vi "Run.vi"(8 "error in (no error)":errorcluster, 11 "TCS in":refnum<class "TCS.lvclass">) -> (0 "error out":errorcluster, 3 "TCS out":refnum<class "TCS.lvclass">)   [LabVIEW 2018, in "TCS.lvclass"]
uses:
  TCS.lvclass
  TCS.lvclass/TCS.ctl
  State Machine/State Machine.lvclass/State Machine.ctl
  State Machine/State Machine.lvclass
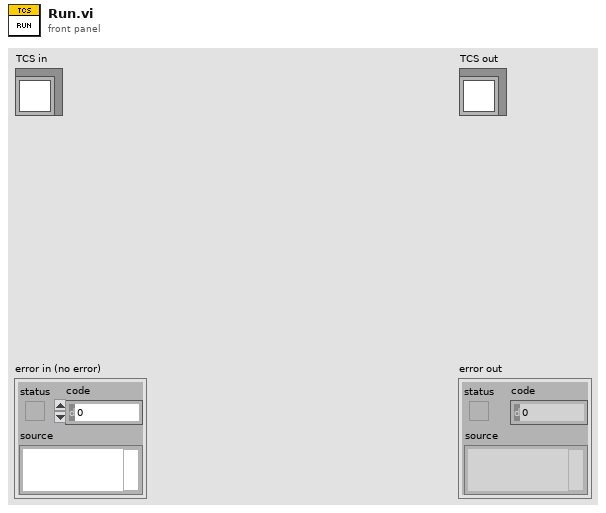
[diagram p1: front panel]
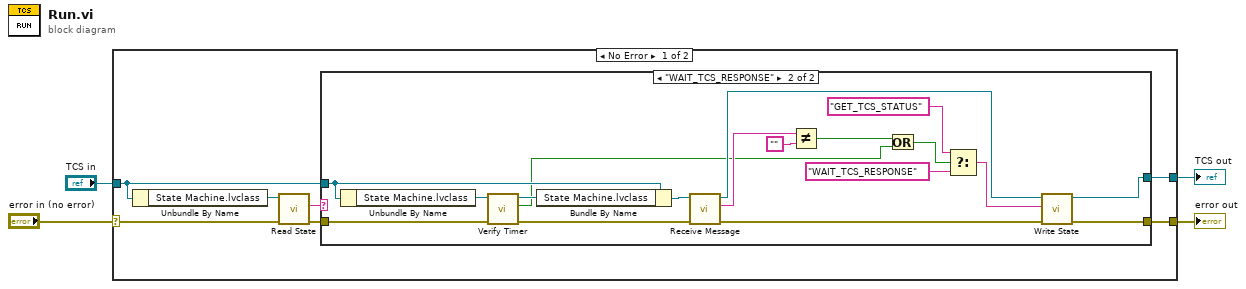
[diagram p0: block diagram]
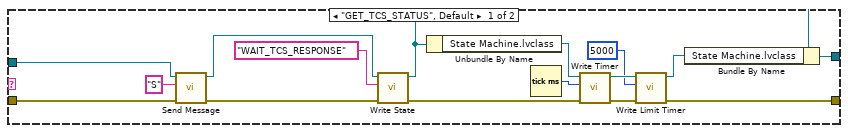
[diagram p2: hidden frame]
diagram:
  n1 = case shown="No Error" "error in (no error)" {
    selector: "error in (no error)" -> [w10 w47]
    tunnel: [w5 w47] -> w3
    tunnel: [w6 w46] -> w1
    tunnel: "TCS in" -> [w8 w46]
    frame No Error {
      n2 = Unbundle By Name(w8) -> ("State Machine.lvclass"=w11:refnum<class "State Machine.lvclass">)
      n3 = call-dynamic "Read State.vi"("error in (no error)"=w10, "State Machine in"=w11) -> ("error out"=w7:errorcluster, "State"=w9:string)  [unwired: 7 in, 1 out]
      n4 = case shown="\"WAIT_TCS_RESPONSE\"" w9 {
        tunnel: w8 -> [w27 w38]
        tunnel: w7 -> [w26 w32]
        tunnel: [w20 w34] -> w6
        tunnel: [w17 w31] -> w5
        frame "GET_TCS_STATUS", Default {
          n5 = call "Send Message.vi"("error in (no error)"=w26, "message"="S", "TCS in"=w27) -> ("error out"=w23:errorcluster, "TCS out"=w24:refnum<class "TCS.lvclass">)  [unwired: 7 in]
          n6 = call "Write State.vi"("error in (no error)"=w23, "State"="WAIT_TCS_RESPONSE" ("message"), "TCS in"=w24) -> ("error out"=w14:errorcluster, "TCS out"=w21:refnum<class "TCS.lvclass">)  [unwired: 7 in]
          n7 = Unbundle By Name(w21) -> ("State Machine.lvclass"=w15:refnum<class "State Machine.lvclass">)
          n8 = Tick Count (ms)() -> (millisecond timer value=w12:u32)
          n9 = call "Write Timer.vi"("error in (no error)"=w14, "Timer"=w12, "State Machine in"=w15) -> ("error out"=w16:errorcluster, "State Machine out"=w19:refnum<class "State Machine.lvclass">)  [unwired: 7 in]
          n10 = call "Write Limit Timer.vi"("error in (no error)"=w16, "Limit Timer"=5000, "State Machine in"=w19) -> ("error out"=w17:errorcluster, "State Machine out"=w18:refnum<class "State Machine.lvclass">)  [unwired: 7 in]
          n11 = Bundle By Name(cluster=w21, "State Machine.lvclass"=w18) -> (w20:refnum<class "TCS.lvclass">)
        }
        frame "WAIT_TCS_RESPONSE" {
          n12 = Unbundle By Name(w38) -> ("State Machine.lvclass"=w37:refnum<class "State Machine.lvclass">)
          n13 = call "Verify Timer.vi"("error in (no error)"=w32, "State Machine in"=w37) -> ("error out"=w33:errorcluster, "time out"=w29:bool, "State Machine out"=w36:refnum<class "State Machine.lvclass">)  [unwired: 7 in]
          n14 = Bundle By Name(cluster=w38, "State Machine.lvclass"=w36) -> (w35:refnum<class "TCS.lvclass">)
          n15 = call "Receive Message.vi"("error in (no error)"=w33, "TCS in"=w35) -> ("error out"=w41:errorcluster, "Rx Message"=w45:string, "TCS out"=w40:refnum<class "TCS.lvclass">)  [unwired: 7 in]
          n16 = Not Equal?(x=w45, y="") -> (x != y?=w30:bool)
          n17 = Or(x=w30, y=w29) -> (x .or. y?=w28:bool)
          n18 = Select(t="GET_TCS_STATUS", s=w28, f="WAIT_TCS_RESPONSE") -> (s? t:f=w39:string)
          n19 = call "Write State.vi"("error in (no error)"=w41, "State"=w39, "TCS in"=w40) -> ("error out"=w31:errorcluster, "TCS out"=w34:refnum<class "TCS.lvclass">)  [unwired: 7 in]
        }
      }
    }
    frame Error {
    }
  }
  "error out" <- w3
  "TCS out" <- w1
